vi "clusters.vi"() -> ()   [LabVIEW 2025]
panel:
  out "Thermometer":dbl
  out "Tank":dbl
  out "Boolean 2":bool
  out "Boolean":bool
  in  "cluster":T1 {"Thermometer" scale=0.0..100.0; "Tank" scale=0.0..10.0}
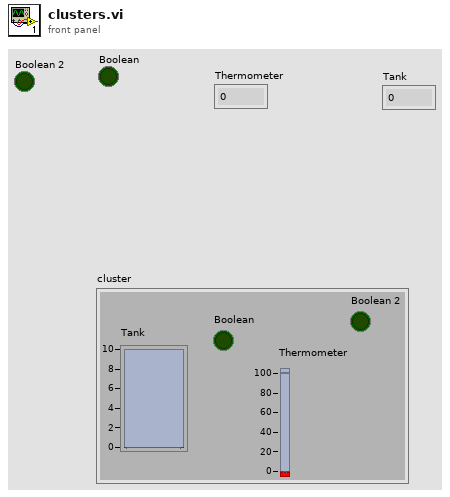
[diagram p1: front panel]
types:
  T1 = cluster{"Boolean":bool, "Boolean 2":bool, "Tank":dbl, "Thermometer":dbl}
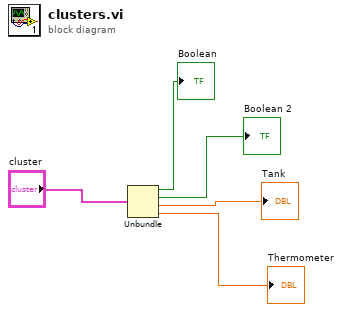
[diagram p0: block diagram]
diagram:
  n1 = Unbundle("cluster") -> ("Boolean"=→"Boolean":bool, "Boolean 2"=→"Boolean 2":bool, "Tank"=→"Tank":dbl, "Thermometer"=→"Thermometer":dbl)
